vi "数组插入组合.vi"(10 "排序后的一维数组":string[](array[string]), 11 "输入数组":string[][](array[string])) -> (3 "输出结果":string[][](array[string]))   [LabVIEW 2016, in "数据传输系统.lvlib"]
uses:
  <userlib>/_OpenG.lib/array/array.llb/Search 1D Array (String)__ogtk.vi
  <userlib>/_OpenG.lib/array/array.llb/Delete Elements from 2D Array (String)__ogtk.vi
panel:
  out "数组":string[][](array[string])
  out "禁用的索引 (列)":i32
  out "Indices of Elements":i32[](array[numeric])
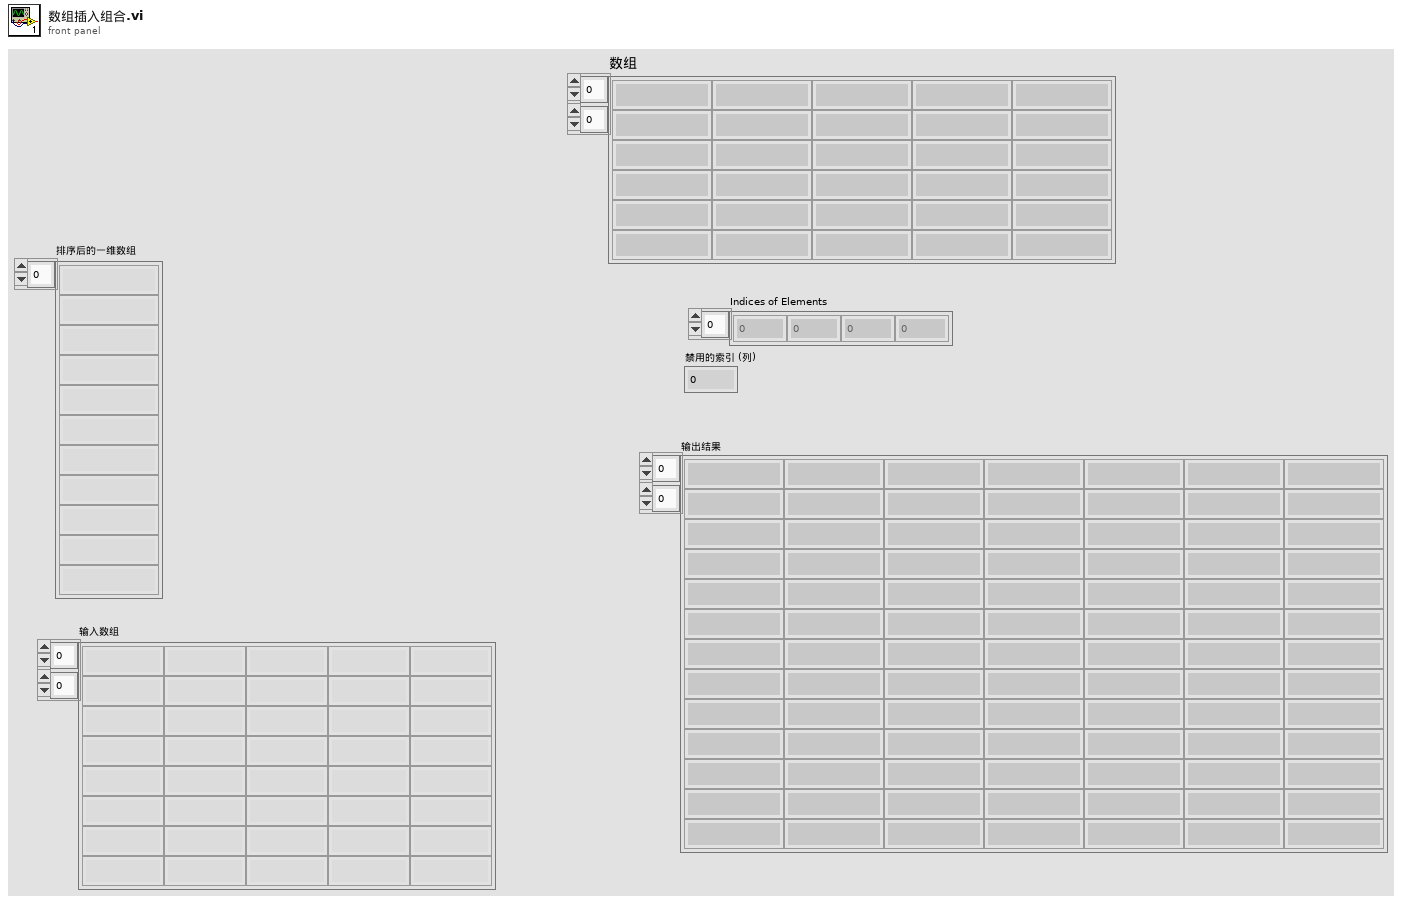
[diagram p1: front panel]
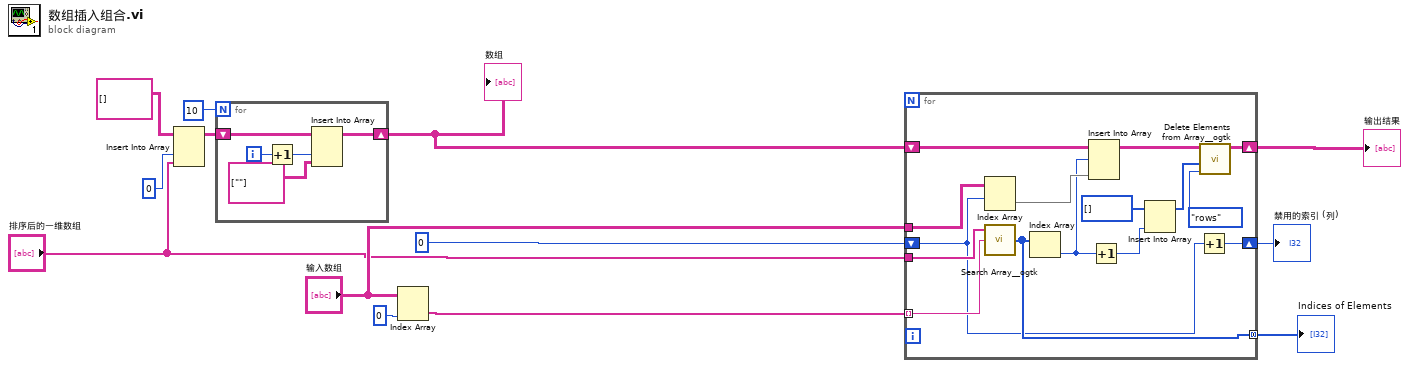
[diagram p0: block diagram]
diagram:
  n1 = Insert Into Array(array=string[][] [], index (col)=0 ("禁用的索引 (列)"), new element="排序后的一维数组") -> (w11:string[][])  [unwired: 1 in]
  n2 = for {
    N: 10 -> [_]
    shift-right: [w17] -> w4
    shift-left: w11 -> [w18]
    i -> [w16]
    n3 = Increment(x=w16) -> (x+1=w15:i32)
    n4 = Insert Into Array(array=w18, index (col)=w15, new element=string[][] [[""]]) -> (w17:string[][])  [unwired: 1 in]
  }
  "数组" <- w4
  n5 = Index Array(array="输入数组", index (col)=0 ("禁用的索引 (列)")) -> (element=w9:string[])  [unwired: 1 in]
  n6 = for {
    tunnel: w9 -> [w33] mode=indexing
    tunnel: "排序后的一维数组" -> [w32]
    tunnel: [w30] -> w8 mode=concatenating
    shift-right: [w24] -> w7
    shift-left: w4 -> [w31]
    shift-right: [w29] -> w6
    shift-left: 0 ("禁用的索引 (列)") -> [w26]
    tunnel: "输入数组" -> [w28]
    n7 = Index Array(array=w28, index (row)=w26) -> (element=w27:string[])  [unwired: 1 in]
    n8 = call-poly <userlib>:"Search Array__ogtk.vi"("Array"=w32, "Element Data"=w33) -> ("Indices of Elements"=w30:i32[])  [unwired: 7 in]
    n9 = Index Array(array=w30) -> (element=w23:i32)  [unwired: 1 in]
    n10 = Insert Into Array(array=w31, index (row)=w23, new element=w27) -> (w25:string[][])  [unwired: 1 in]
    n11 = Increment(x=w23) -> (x+1=w20:i32)
    n12 = Insert Into Array(array=i32[] [] ("indices"), new element=w20) -> (w21:i32[])  [unwired: 1 in]
    n13 = Increment(x=w26) -> (x+1=w29:i32)
    n14 = call-poly <userlib>:"Delete Elements from Array__ogtk.vi"("delete (rows or columns)"=enum16{"rows", "columns"}."rows", "indices"=w21, "array"=w25) -> ("array w/ subset deleted"=w24:string[][])  [unwired: 7 in, 1 out]
  }
  "Indices of Elements" <- w8
  "输出结果" <- w7
  "禁用的索引 (列)" <- w6
